vi "RR_scripting.vi"   [LabVIEW 2024]
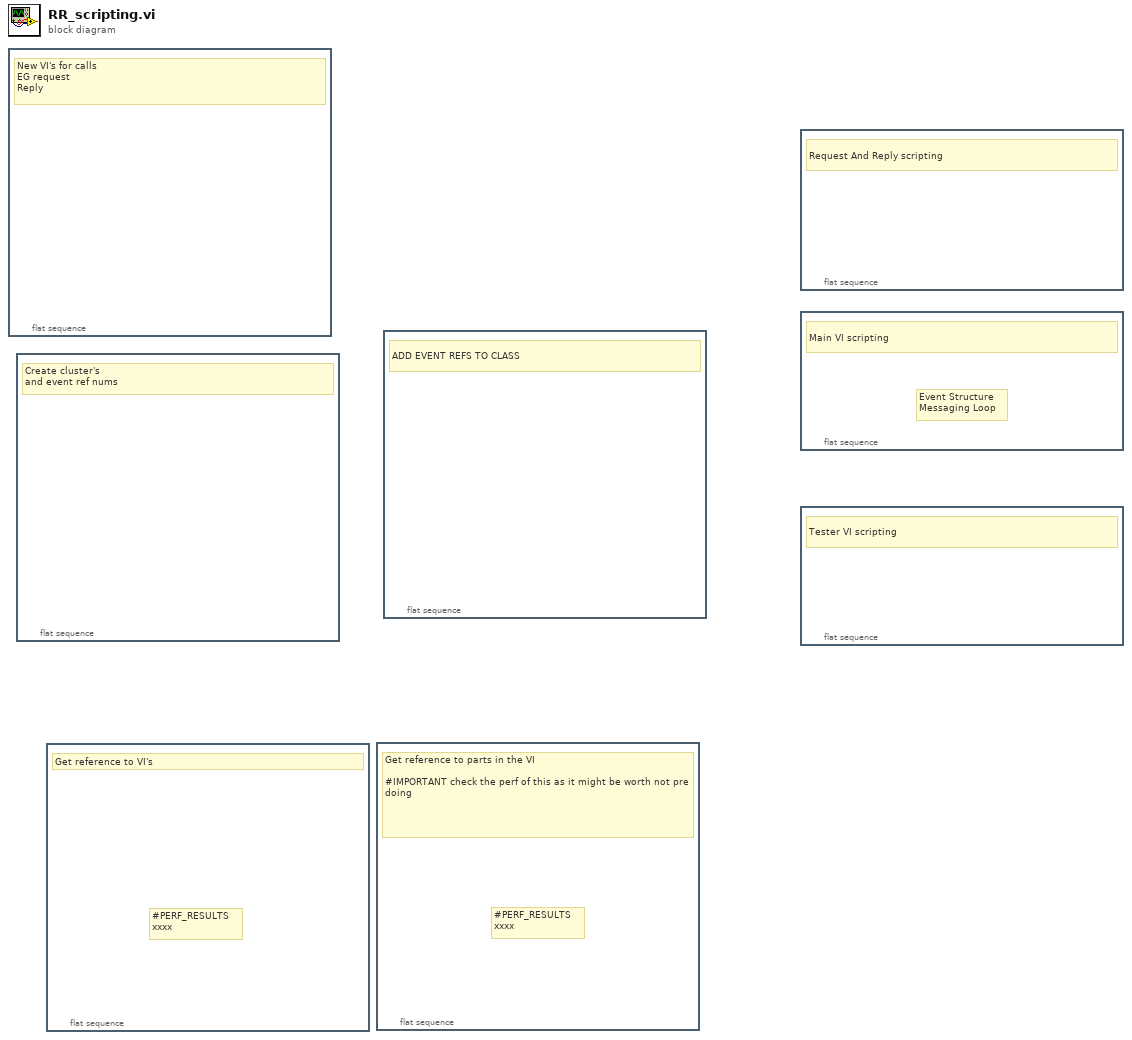
[diagram p0: block diagram]
diagram:
  n1 = flat-sequence {
    frame #0 {
      # "New VI's for calls\nEG request\nReply"
    }
  }
  n2 = flat-sequence {
    frame #0 {
      # "Create cluster's\nand event ref nums"
    }
  }
  n3 = flat-sequence {
    frame #0 {
      # "#PERF_RESULTS\nxxxx"
      # "Get reference to VI's"
    }
  }
  n4 = flat-sequence {
    frame #0 {
      # "#PERF_RESULTS\nxxxx"
      # "Get reference to parts in the VI\n\n#IMPORTANT check the perf of this as it might be worth not pre doing"
    }
  }
  n5 = flat-sequence {
    frame #0 {
      # "ADD EVENT REFS TO CLASS"
    }
  }
  n6 = flat-sequence {
    frame #0 {
      # "Request And Reply scripting"
    }
  }
  n7 = flat-sequence {
    frame #0 {
      # "Event Structure\nMessaging Loop"
      # "Main VI scripting"
    }
  }
  n8 = flat-sequence {
    frame #0 {
      # "Tester VI scripting"
    }
  }
